vi "ReadTDMSFileFromDataLogConfiguration.vi"(8 "error in (no error)":errorcluster, 11 "Data Log File Configuration":T1) -> (0 "error out":errorcluster, 2 "data":waveform(dbl)[](array[waveform]), 3 "channel name(s) out":string[](array[string]))   [LabVIEW 2016, in "VeriStandTestUtilities.lvlib"]
uses:
  VeriStandTestUtilities/VeriStandTestUtilities.lvlib
  <vilib>/NI Veristand/Execution/Workspace/LogFileConfiguration.ctl
  <vilib>/NI Veristand/Execution/Workspace/LogFileTriggerConfiguration.ctl
  <vilib>/NI Veristand/Execution/Workspace/LogFileTriggerType.ctl
  <vilib>/NI Veristand/Execution/Workspace/LogProperty.ctl
  <vilib>/NI Veristand/Execution/Workspace/LogChannelConfiguration.ctl
  <vilib>/NI VeriStand/Execution/Workspace/NI_VS Workspace ExecutionAPI.lvlib
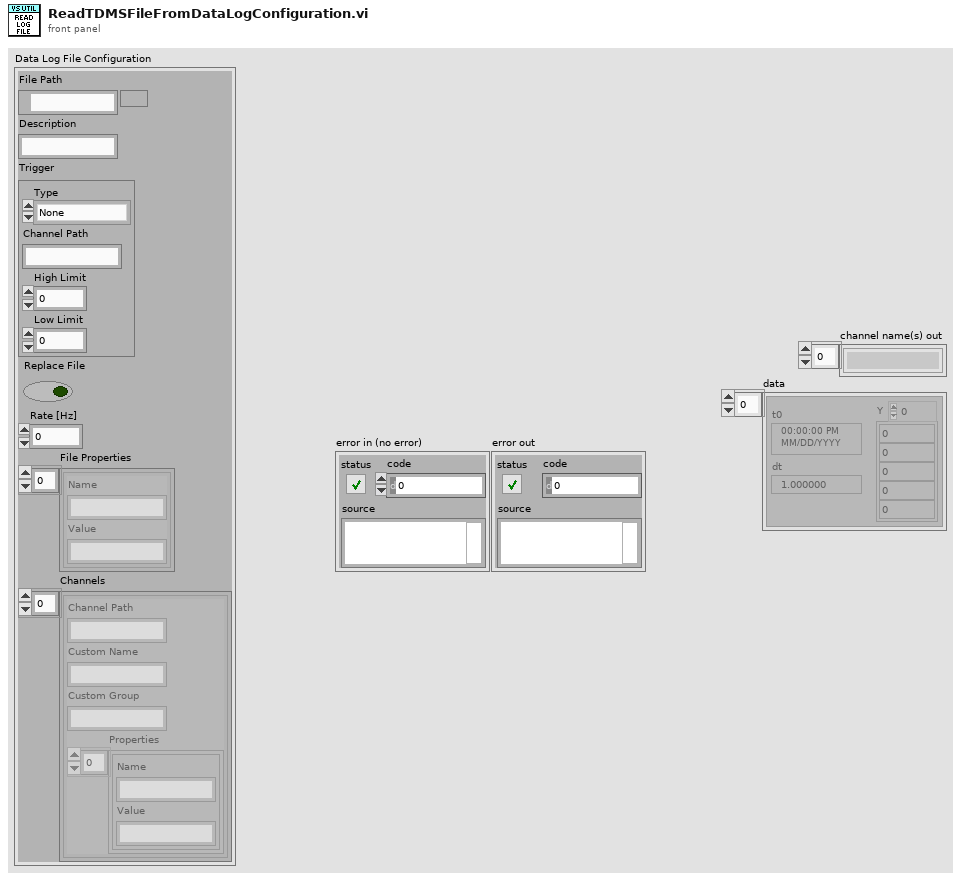
[diagram p1: front panel]
types:
  T1 = typedef "NI_VS Workspace ExecutionAPI.lvlib/LogFileConfiguration.ctl" = cluster{"File Path":path, "Description":string, "Trigger":T2, "Replace File":bool, "Rate [Hz]":dbl, "File Properties":T4[], "Channels":T5[]}
  T2 = typedef "NI_VS Workspace ExecutionAPI.lvlib/LogFileTriggerConfiguration.ctl" = cluster{"Type":T3, "Channel Path":string, "High Limit":dbl, "Low Limit":dbl}
  T3 = typedef "NI_VS Workspace ExecutionAPI.lvlib/LogFileTriggerType.ctl" = enum16{"None", "In Limits", "Out of Limits"}
  T4 = typedef "NI_VS Workspace ExecutionAPI.lvlib/LogProperty.ctl" = cluster{"Name":string, "Value":string}
  T5 = typedef "NI_VS Workspace ExecutionAPI.lvlib/LogChannelConfiguration.ctl" = cluster{"Channel Path":string, "Custom Name":string, "Custom Group":string, "Properties":T4[]}
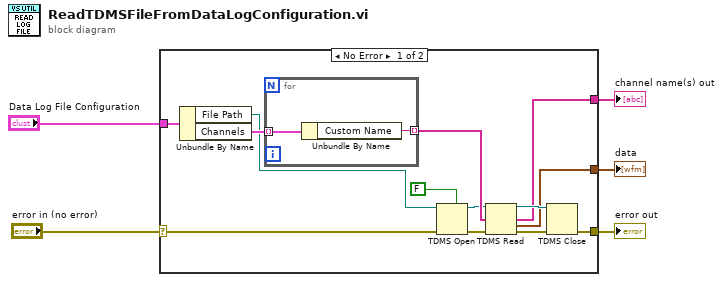
[diagram p0: block diagram]
diagram:
  n1 = case shown="No Error" "error in (no error)" {
    selector: "error in (no error)" -> [w9 w21]
    tunnel: "Data Log File Configuration" -> [w11 _]
    tunnel: [w10 _] -> w4
    tunnel: [w8 w21] -> w2
    tunnel: [w7 _] -> w1
    frame No Error {
      n2 = Unbundle By Name(w11) -> ("File Path"=w14:path, "Channels"=w15:T5[])
      n3 = for {
        tunnel: w15 -> [w20] mode=indexing
        tunnel: [w19] -> w16 mode=indexing
        n4 = Unbundle By Name(w20) -> ("Custom Name"=w19:string)
      }
      n5 = TDMS Open(5:FALSE ("create index file? (T)"), 8:w9, 11:w14) -> (0:w13:errorcluster, 3:w12:refnum<k34>)  [unwired: 4 in]
      n6 = TDMS Read(0:w12, 7:w16, 11:w13) -> (4:w18:refnum<k34>, 8:w10:string[], 10:w7:waveform(dbl)[], 15:w17:errorcluster)  [unwired: 5 in, 2 out]
      n7 = TDMS Close(8:w17, 11:w18) -> (0:w8:errorcluster)  [unwired: 1 out]
    }
    frame Error {
    }
  }
  "channel name(s) out" <- w4
  "error out" <- w2
  "data" <- w1
